vi "libssh2_agent_userauth.vi"(8 "error in (no error)":errorcluster, 9 "public key":T1, 10 "username":string, 11 "agent":T2) -> (0 "error out":errorcluster, 2 "authenticated":bool)   [LabVIEW 2013, in "libssh2.lvlib"]
doc: "Authenticate a session with a public key from an SSH agent."
uses:
  libssh2.lvlib
  Agent Refnum.ctl
  Agent Public Key Refnum.ctl
  Not An Agent.vi
  <vilib>/Utility/error.llb/Error Cluster From Error Code.vi
  Not An Agent Public Key.vi
  Global Settings.vi
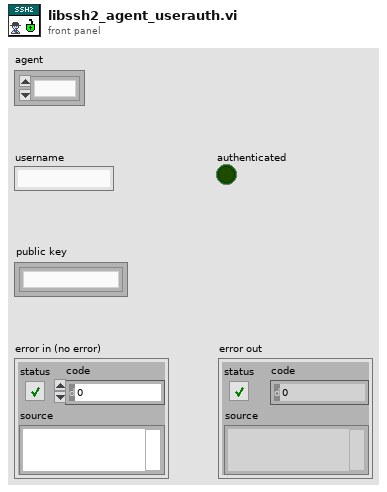
[diagram p1: front panel]
types:
  T1 = typedef "libssh2.lvlib/Agent Public Key Refnum.ctl" = refnum<k1>
  T2 = typedef "libssh2.lvlib/Agent Refnum.ctl" = refnum<k1>
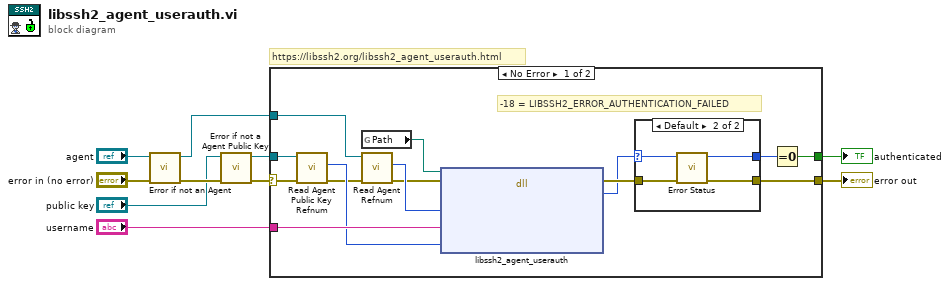
[diagram p0: block diagram]
diagram:
  # "https://libssh2.org/libssh2_agent_userauth.html"
  n1 = call "Error if not an Agent.vi"("error in (no error)"="error in (no error)", "agent"="agent") -> ("error out"=w6:errorcluster, "agent out"=w4:T2)  [unwired: 8 in]
  n2 = call "Error if not a Agent Public Key.vi"("error in (no error)"=w6, "agent public key"="public key") -> ("error out"=w3:errorcluster, "agent public key out"=w1:T1)  [unwired: 8 in]
  n3 = case shown="No Error" w3 {
    selector: w3 -> [w12 w31]
    tunnel: [w24 w31] -> w10
    tunnel: w1 -> [w22 _]
    tunnel: "username" -> [w23 _]
    tunnel: [w21 _] -> w7
    tunnel: w4 -> [w20 _]
    frame No Error {
      # "-18 = LIBSSH2_ERROR_AUTHENTICATION_FAILED"
      n4 = call "Read Agent Public Key Refnum.vi"("error in (no error)"=w12, "agent public key"=w22) -> ("error out"=w11:errorcluster, "libssh2_agent_publickey*"=w16:u64)  [unwired: 8 in]
      n5 = global read "Global Settings.vi" "Path"() -> (w19:path)
      n6 = call "Read Agent Refnum.vi"("error in (no error)"=w11, "agent"=w20) -> ("error out"=w13:errorcluster, "LIBSSH2_AGENT*"=w18:u64)  [unwired: 8 in]
      n7 = dll-call lib="?" fn="libssh2_agent_userauth"(path in=w19, error in=w13, "agent"=w18, "username"=w23, "identity"=w16) -> (error out=w17:errorcluster, "return value"=w15:i32)  [unwired: 4 in, 1 out]
      n8 = case shown="Default" w15 {
        selector: w15 -> [w25 w28]
        tunnel: w17 -> [w26 w30]
        tunnel: [w26 w29] -> w24
        tunnel: [w25 w27] -> w14
        frame -18 {
        }
        frame Default {
          n9 = call "Error Status.vi"("error in (no error)"=w30, "return value"=w28) -> ("error out"=w29:errorcluster, "return value out"=w27:i32)  [unwired: 8 in]
        }
      }
      n10 = Equal To 0?(x=w14) -> (x = 0?=w21:bool)
    }
    frame Error {
    }
  }
  "error out" <- w10
  "authenticated" <- w7
